vi "DSF.Engine.Status.Framework.Performance.Set Rx Start Time.vi"(10 "Rx start time":u32 format="%d us", 11 "Framework Performance in":refnum<class "DSF.Engine.Status.Framework.Performance.lvclass">) -> (3 "Framework Performance out":refnum<class "DSF.Engine.Status.Framework.Performance.lvclass">)   [LabVIEW 2017, in "Data Sharing Framework Engine.lvlib" / "DSF.Engine.Status.Framework.Performance.lvclass"]
uses:
  DSF.Engine.Status.Framework.Performance.lvclass
  DSF.Engine.Status.Framework.Performance.lvclass/DSF.Engine.Status.Framework.Performance.ctl
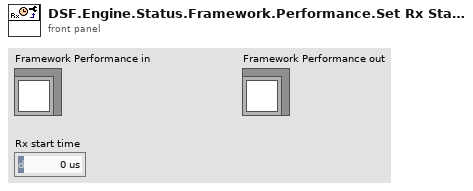
[diagram p1: front panel]
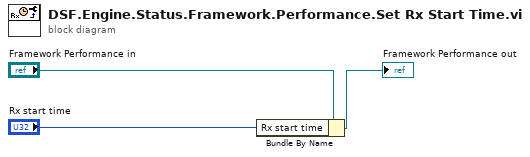
[diagram p0: block diagram]
diagram:
  n1 = Bundle By Name(cluster="Framework Performance in", "Rx start time"="Rx start time") -> (→"Framework Performance out":refnum<class "DSF.Engine.Status.Framework.Performance.lvclass">)
